vi "Actor Core.vi"(8 "error in":errorcluster, 11 "Nested in":refnum<class "Network Management UI.lvclass">) -> (0 "error out":errorcluster, 3 "Actor out":refnum<class "Actor.lvclass">)   [LabVIEW 2024, in "Network Management UI.lvlib" / "Network Management UI.lvclass"]
doc: "(<B>Filename</B>: Actor Framework.lvlib:Actor.lvclass:Actor Core.vi)\n\nReceives messages to the actor, reacts to them, and initiates any error handling that may shut the actor down.\n\nDescendant classes may override this VI to append parallel tasks for the actor to complete while it handles messages. Overrides use the Call Parent Method node."
uses:
  Network Management UI.lvclass
  Network Management UI.lvclass/Network Management UI.ctl
  <vilib>/ActorFramework/Stop Msg/Stop Msg.lvclass
  <vilib>/MGI/Panel Manager/Panel Actor/Panel Actor/Panel Actor.lvclass
  <vilib>/ActorFramework/Actor/Actor.lvclass
  Example/Interactor Messages/Set Heartbeat Producer Msg/Set Heartbeat Producer Msg.lvclass
  Example/Interactor Messages/Add Expected Heartbeat Msg/Add Expected Heartbeat Msg.lvclass
  C:/Program Files/National Instruments/LabVIEW 2025/vi.lib/MGI/Panel Manager/Panel Actor/Panel Actor/Panel Actor.lvclass
  C:/Program Files/National Instruments/LabVIEW 2025/vi.lib/ActorFramework/Actor/Actor.lvclass
  D:/git/CANopen-XNET/Network Management UI/Network Management UI.lvclass
panel:
  in  "Tab Control":enum32{"Heartbeat", "Page 2"}(tab)
  in  "Set Expected Heartbeat Button 2":bool
  in  "Set Expected Heartbeat Button":bool
  in  "Timeout":u16 format="%d ms"
  in  "Period":u16 format="%d ms"
  in  "Node-ID":u8
  in  "Heartbeat Production":u32 format="%d ms"
  out "Expected Heartbeats":T1(c390)
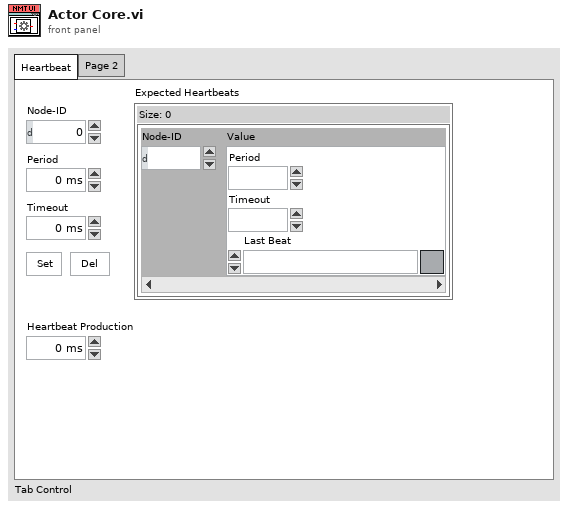
[diagram p1: front panel]
types:
  T1 = map{u8, cluster{"Period":u16, "Timeout":u16, "Last Beat":timestamp}}
  T2 = cluster{"Pnl Actor":refnum<event-registration>, "Event Registration Refnum":refnum<event-registration>}
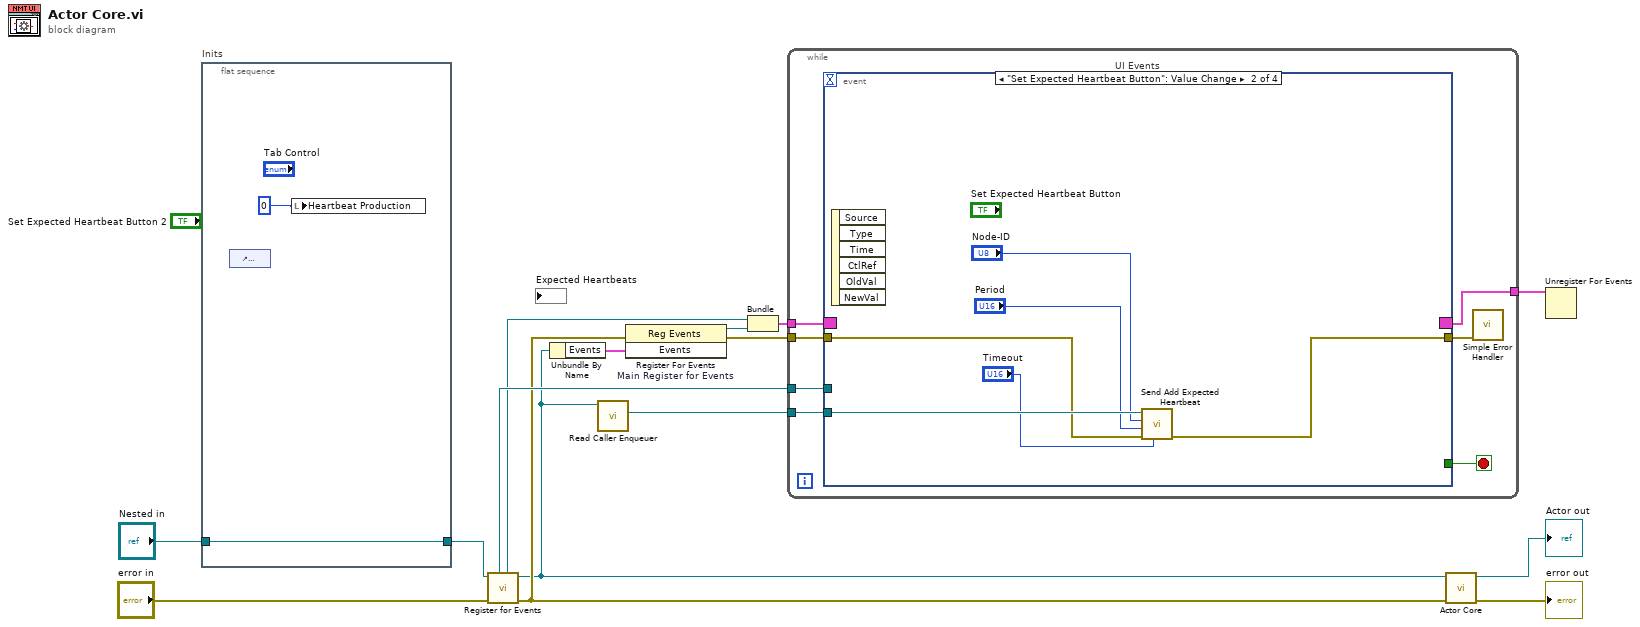
[diagram p0: block diagram]
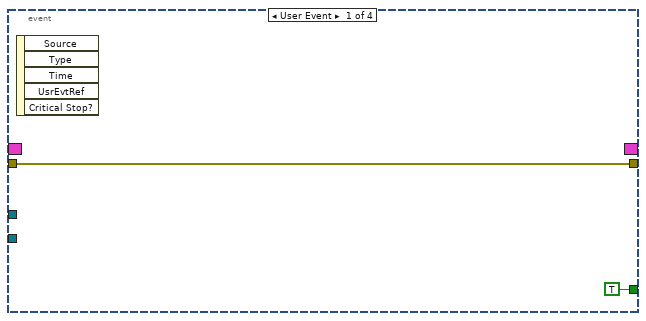
[diagram p2: hidden frame]
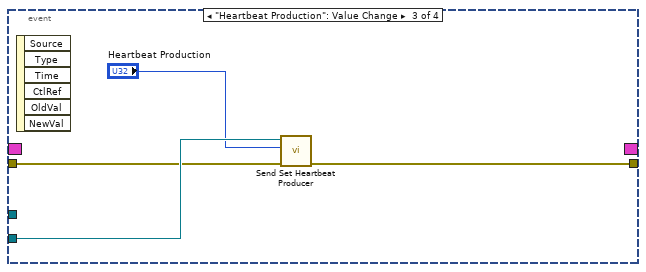
[diagram p3: hidden frame]
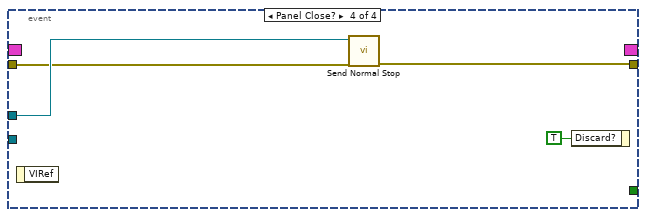
[diagram p4: hidden frame]
diagram:
  n1 = flat-sequence "Inits" {
    tunnel: "Nested in" -> [w17]
    tunnel: [w17] -> w5
    frame #0 {
      n2 = control-ref of="Expected Heartbeats"() -> ()  [unwired: 1 out]
      n3 = local write "Heartbeat Production"(u32 0 ("Heartbeat Production")) -> ()
    }
  }
  n4 = call <vilib>:"Register for Events.vi"("Error In"="error in", "Panel Actor in"=w5) -> ("Error Out"=w8:errorcluster, "Panel Actor out"=w2:refnum<class "Network Management UI.lvclass">, "Pnl Actor"=w4:refnum<event-registration>, "Self Enqueuer"=w10:refnum<class "Message Enqueuer.lvclass">)  [unwired: 6 in]
  n5 = Unbundle By Name(w2) -> ("Events"=w13:cluster{"None":refnum<user-event>})
  n6 = call <vilib>:"Read Caller Enqueuer.vi"("Actor"=w2) -> ("Caller Enqueuer"=w1:refnum<class "Message Enqueuer.lvclass">)  [unwired: 10 in]
  n7 = register-events "Main Register for Events"(error in=w8, w13) -> (reference out=w3:refnum<event-registration>, error out=w7:errorcluster)  [unwired: 1 in]
  n8 = Bundle("Pnl Actor"=w4, "Event Registration Refnum"=w3) -> (w9:T2)  [unwired: 1 in]
  n9 = while {
    tunnel: w9 -> [w24]
    tunnel: [w22] -> w12
    tunnel: w10 -> [w21]
    tunnel: w7 -> [w20]
    tunnel: w1 -> [w19]
    stop <- w23 stop-if-true
    n10 = event "UI Events" shown="[1] \"Set Expected Heartbeat Button\": Value Change" {
      selector: w24 -> [_ _ _ _]
      dyn-events: [_ _ _ _] -> w22
      timeout: _ -> [_ _ _ _]
      tunnel: [TRUE _ _ _] -> w23
      tunnel: w21 -> [_ _ _ w39]
      tunnel: w20 -> [w25 w27 w34 w38]
      tunnel: w19 -> [_ w32 w36 _]
      tunnel: [w25 w28 w33 w37] -> w18
      event User Event {
        n11 = event-data() -> ()  [unwired: 1 in, 5 out]
      }
      event "Set Expected Heartbeat Button": Value Change {
        n12 = event-data() -> ()  [unwired: 1 in, 6 out]
        n13 = call "Send Add Expected Heartbeat.vi"("Timeout"="Timeout", "error in (no error)"=w27, "Period"="Period", "Node-ID"="Node-ID", "Message Enqueuer"=w32) -> ("error out"=w28:errorcluster)  [unwired: 5 in, 1 out]
      }
      event "Heartbeat Production": Value Change {
        n14 = event-data() -> ()  [unwired: 1 in, 6 out]
        n15 = call "Send Set Heartbeat Producer.vi"("error in (no error)"=w34, "Heartbeat Production"="Heartbeat Production", "Message Enqueuer"=w36) -> ("error out"=w33:errorcluster)  [unwired: 7 in, 1 out]
      }
      event Panel Close? {
        n16 = event-data() -> ()  [unwired: 1 in, 1 out]
        n17 = call <vilib>:"Send Normal Stop.vi"("error in (no error)"=w38, "Message Enqueuer"=w39) -> ("error out"=w37:errorcluster)  [unwired: 9 in]
        n18 = event-data("Discard?"=TRUE) -> ()  [unwired: 1 in, 1 out]
      }
    }
    n19 = call <vilib>:"Simple Error Handler.vi"("error in (no error)"=w18) -> ()  [unwired: 4 in, 5 out]
  }
  n20 = call-parent "Actor Core.vi"("error in"=w8, "Panel Actor in"=w2) -> ("error out"=→"error out":errorcluster, "Actor out"=→"Actor out":refnum<class "Actor.lvclass">)  [unwired: 8 in]
  n21 = Unregister For Events(event registration refnum=w12) -> ()  [unwired: 1 in, 1 out]
